vi "Get 2D I64.vi"(7 "key description":string, 8 "sections":string[](array[string]), 9 "numeric":i64[][](array[numeric]), 11 "info data":string) -> (0 "sections out":string[](array[string]), 1 "key found?":bool, 2 "value":i64[][](array[numeric]), 3 "info data out":string)   [LabVIEW 2020, in "infolib.lvlib"]
doc: "Reads matrix of 64 bit integers. If section is entered it searches the key in the section(s).\nInput 'numeric' can be used to set default value.\nIf key is not found, the output value is equal to 'numeric' input.\nIf key is found, and element of matrix cannot be converted into data type, the default value of output matrix element is based on:\n- first element of 'numeric' input if available\n- otherwise maximum of I64 is used."
uses:
  infolib.lvlib
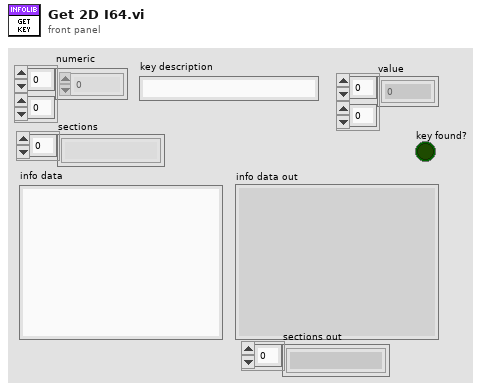
[diagram p1: front panel]
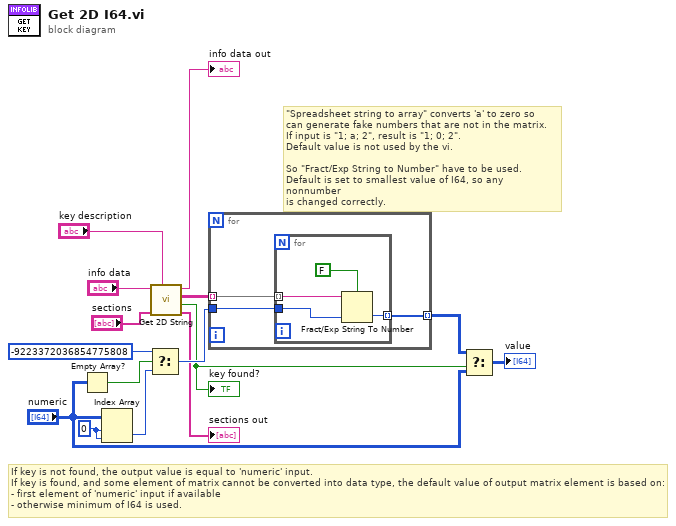
[diagram p0: block diagram]
diagram:
  w13 = 0 ("index (row)")
  # "If key is not found, the output value is equal to 'numeric' input.\nIf key is found, and some element of matrix cannot be converted into data type, the default value of output matrix element is based on:\n- first element of 'numeric' input if available\n- otherwise minimum of I64 is used."
  # "\"Spreadsheet string to array\" converts 'a' to zero so\ncan generate fake numbers that are not in the matrix.\nIf input is \"1; a; 2\", result is \"1; 0; 2\".\nDefault value is not used by the vi.\n\nSo \"Fract/Exp String to Number\" have to be used.\nDefault is set to smallest value of I64, so any nonnumber\nis changed correctly."
  n1 = Empty Array?(array="numeric") -> (empty?=w11:bool)
  n2 = Index Array(array="numeric", index (row)=w13, index (col)=w13) -> (element=w12:i64)
  n3 = Select(t=i64 -9223372036854775808 ("default (0 DBL)"), s=w11, f=w12) -> (s? t:f=w8:i64)
  n4 = call "Get 2D String.vi"("key description"="key description", "sections"="sections", "info data"="info data") -> ("sections out"=→"sections out":string[], "key found?"=w2:bool, "value"=w1:string[][], "info data out"=→"info data out":string)  [unwired: 5 in]
  "key found?" <- w2
  n5 = for {
    tunnel: w1 -> [w18] mode=indexing
    tunnel: [w17] -> w14 mode=indexing
    tunnel: w8 -> [w16]
    n6 = for {
      tunnel: w18 -> [w21] mode=indexing
      tunnel: [w20] -> w17 mode=indexing
      tunnel: w16 -> [w19]
      n7 = Fract/Exp String To Number(use system decimal point (T)=FALSE, string=w21, default (0 dbl)=w19) -> (number=w20:i64)  [unwired: 1 in, 1 out]
    }
  }
  n8 = Select(t=w14, s=w2, f="numeric") -> (s? t:f=→"value":i64[][])
